vi "Pk-Pk to RMS.vi"(1 "pk-pk":dbl=2.828 format="%.3f") -> (0 "RMS":dbl=nan format="%.3f")   [LabVIEW 2010]
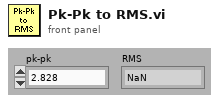
[diagram p1: front panel]
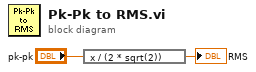
[diagram p0: block diagram]
diagram:
  n1 = expression code="x / (2 * sqrt(2))"("pk-pk") -> (→"RMS":dbl)
